vi "Analysis.Measurement, Build Dimension Info_V3.vi"(6 "UL":string, 8 "LL":string, 9 "Value":string, 10 "Name":string, 11 "MeasDims_In":variant) -> (2 "Added":bool, 3 "MeasDims_Out":variant)   [LabVIEW 2024]
uses:
  Analysis.Measurement Limit Info.ctl
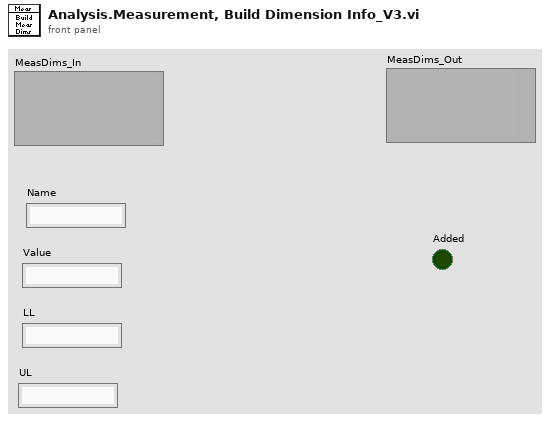
[diagram p1: front panel]
types:
  T1 = typedef "Analysis.Measurement Limit Info.ctl" = cluster{"Name":string, "Numeric":bool, "LL":dbl, "LL_En":bool, "UL":dbl, "UL_En":bool, "Units":string}
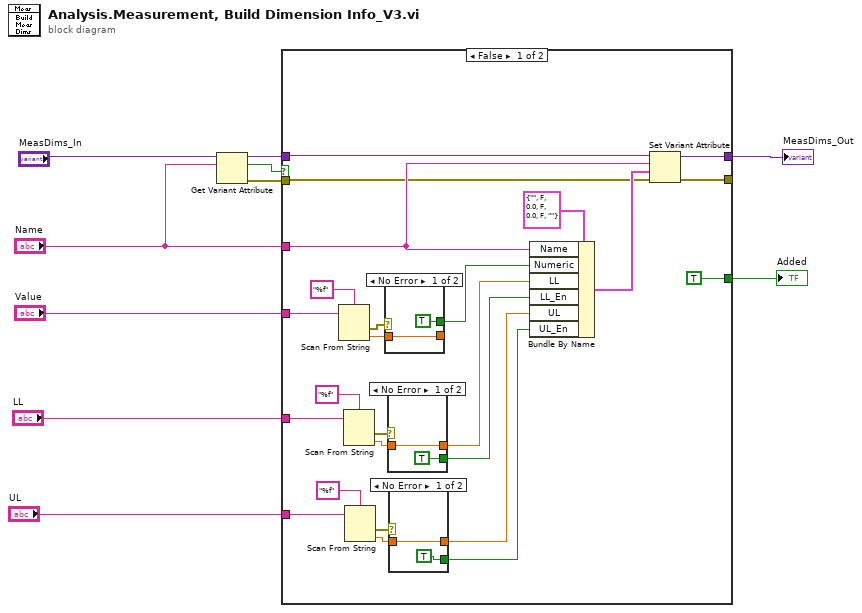
[diagram p0: block diagram]
diagram:
  n1 = Get Variant Attribute(Variant="MeasDims_In", name="Name") -> (duplicate Variant=w8:variant, found=w9:bool, error out=w1:errorcluster)  [unwired: 2 in, 1 out]
  n2 = case shown="False" w9 {
    tunnel: w8 -> [w35 w42]
    tunnel: [w32 w42] -> w7
    tunnel: "Name" -> [w33 _]
    tunnel: [TRUE _] -> w5
    tunnel: "Value" -> [w28 _]
    tunnel: "LL" -> [w25 _]
    tunnel: "UL" -> [w24 _]
    tunnel: w1 -> [w11 _]
    tunnel: [w12 _] -> _
    frame False {
      n3 = Scan From String(format string="%f", input string=w28) -> (error out=w23:errorcluster, output 1=w22:dbl)  [unwired: 3 in, 2 out]
      n4 = Scan From String(format string="%f", input string=w25) -> (error out=w21:errorcluster, output 1=w20:dbl)  [unwired: 3 in, 2 out]
      n5 = Scan From String(format string="%f", input string=w24) -> (error out=w19:errorcluster, output 1=w18:dbl)  [unwired: 3 in, 2 out]
      n6 = case shown="No Error" w23 {
        tunnel: w22 -> [w41 _]
        tunnel: [w41 _] -> _
        tunnel: [TRUE _] -> w15
        frame No Error {
        }
        frame Error {
        }
      }
      n7 = case shown="No Error" w21 {
        tunnel: w20 -> [w39 _]
        tunnel: [w39 _] -> w17
        tunnel: [TRUE _] -> w14
        frame No Error {
        }
        frame Error {
        }
      }
      n8 = case shown="No Error" w19 {
        tunnel: w18 -> [w37 _]
        tunnel: [w37 _] -> w16
        tunnel: [TRUE _] -> w13
        frame No Error {
        }
        frame Error {
        }
      }
      n9 = Bundle By Name(cluster=T1 {"Name"="", "Numeric"=FALSE, "LL"=0.0, "LL_En"=FALSE, "UL"=0.0, "UL_En"=FALSE, "Units"=""} ("Measurement Dimension"), "Name"=w33, "Numeric"=w15, "LL"=w17, "LL_En"=w14, "UL"=w16, "UL_En"=w13) -> (w30:T1)
      n10 = Set Variant Attribute(Variant=w35, name=w33, value=w30, error in=w11) -> (Variant out=w32:variant, error out=w12:errorcluster)  [unwired: 1 out]
    }
    frame True {
    }
  }
  "MeasDims_Out" <- w7
  "Added" <- w5
